vi "pcfs_create_stop_queue.vi"(8 "error in (no error)":errorcluster, 11 "scan_panel in":refnum<class "pcfs.lvclass">) -> (0 "error out":errorcluster, 2 "stop_queue":refnum<queue>, 3 "scan_panel out":refnum<class "pcfs.lvclass">)   [LabVIEW 2015, in "pcfs.lvclass"]
uses:
  pcfs.lvclass
  pcfs.lvclass/pcfs.ctl
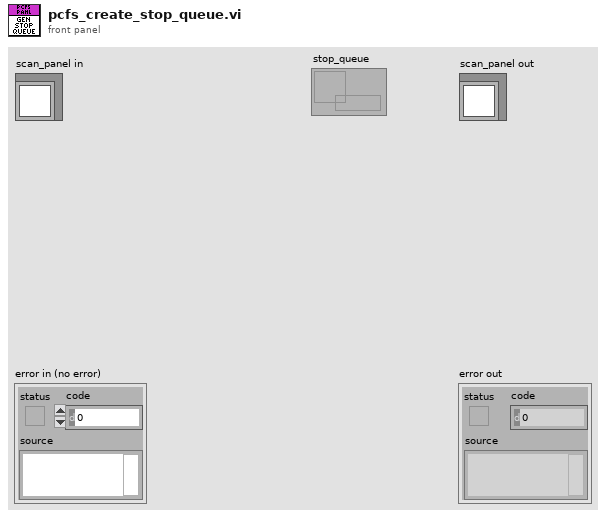
[diagram p1: front panel]
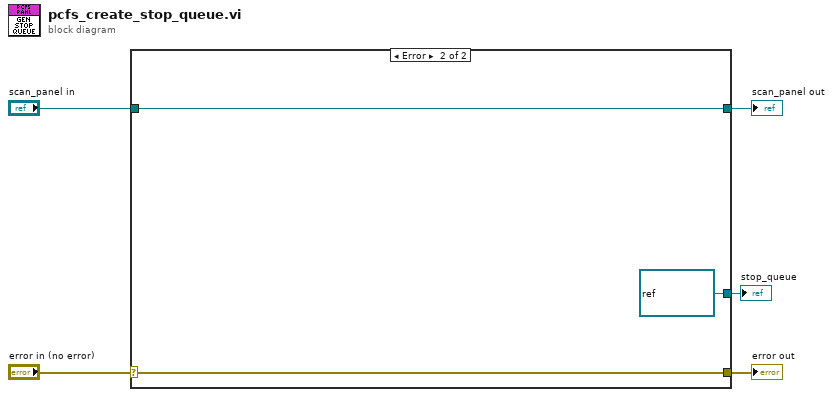
[diagram p0: block diagram]
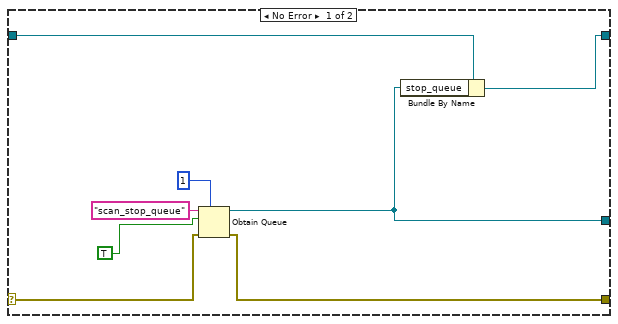
[diagram p2: hidden frame]
diagram:
  n1 = case shown="Error" "error in (no error)" {
    selector: "error in (no error)" -> [w11 w16]
    tunnel: [w8 w16] -> w4
    tunnel: [w7 w15] -> w2
    tunnel: "scan_panel in" -> [w9 w15]
    tunnel: [w6 refnum<queue> refnum ("queue out")] -> w1
    frame No Error {
      n2 = Obtain Queue(max queue size (-1, unlimited)=1, name (unnamed)="scan_stop_queue", element data type=TRUE, error in (no error)=w11) -> (queue out=w6:refnum<queue>, error out=w8:errorcluster)  [unwired: 1 in, 1 out]
      n3 = Bundle By Name(cluster=w9, "stop_queue"=w6) -> (w7:refnum<class "pcfs.lvclass">)
    }
    frame Error {
    }
  }
  "error out" <- w4
  "scan_panel out" <- w2
  "stop_queue" <- w1
